vi "CR-SaveImageCCD3暂存.vi"(6 "类型":string(combo)="Front conveyor", 8 "error in (no error)":errorcluster, 9 "Image in":T1(plugin-control), 10 "布尔":bool=TRUE, 11 "基路径":path) -> (0 "error out":errorcluster)   [LabVIEW 2017]
panel:
  out "日期/时间字符串":string
  in  "CCD Name":string(combo)="CCD3"
  out "连接的字符串":string
  # "D:\\Data\\History Image\\20190228\\CCD3\\Image"
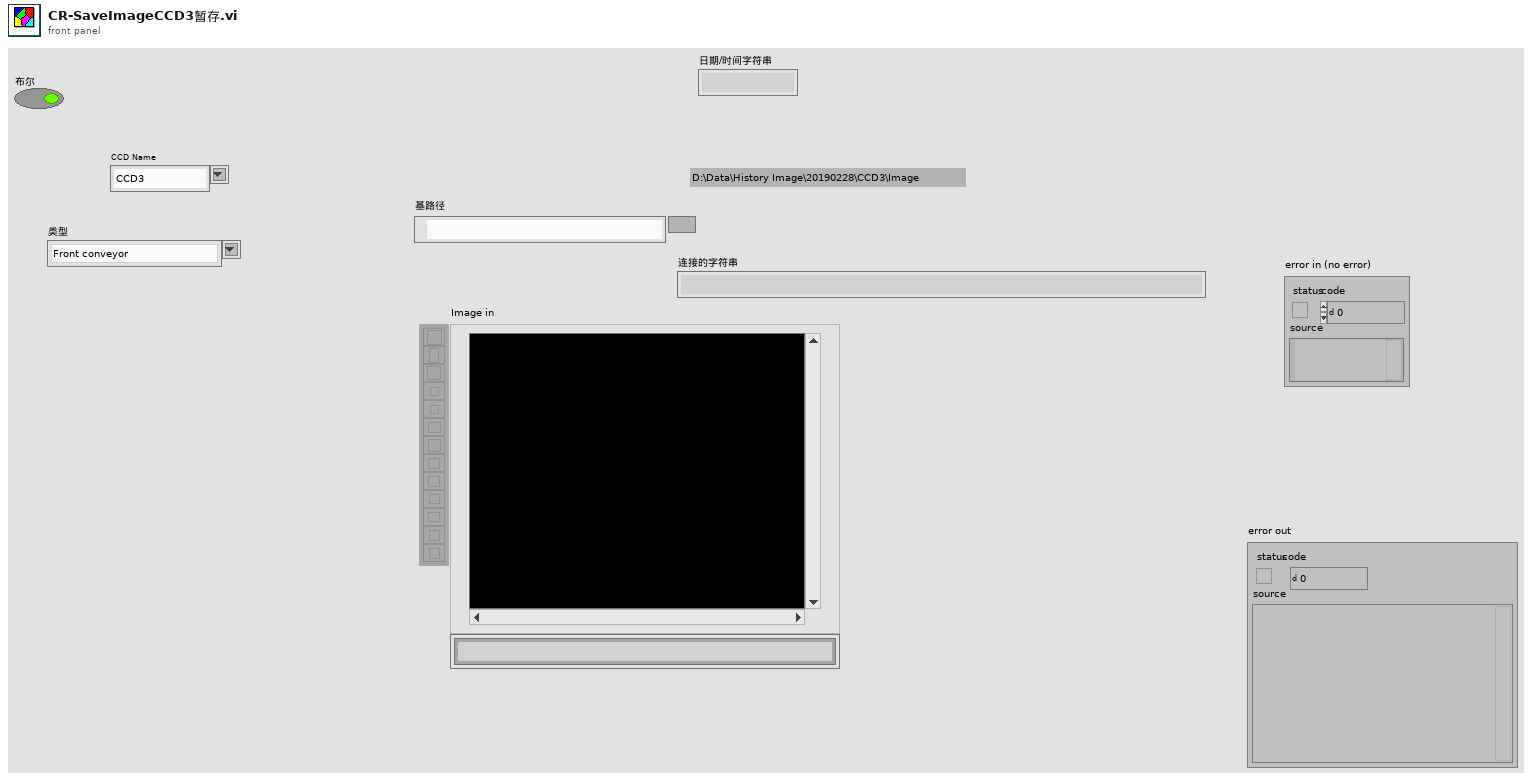
[diagram p1: front panel]
types:
  T1 = typedef "IMAQ Image.ctl" = refnum<image>
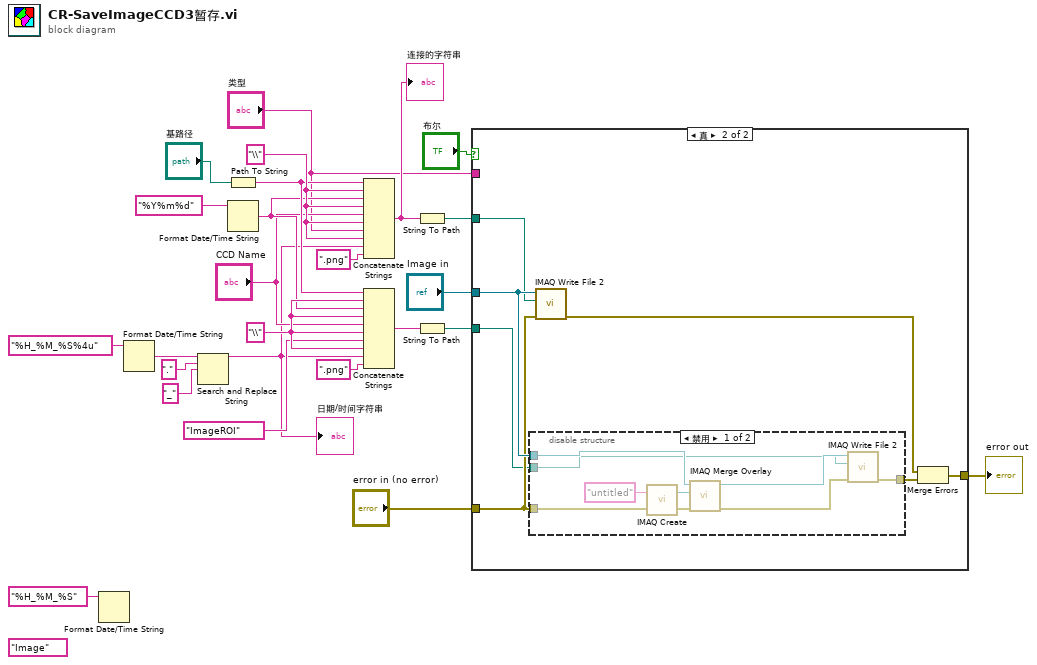
[diagram p0: block diagram]
diagram:
  (unwired) "Image" ("类型")
  w14 = "\\" ("字符串")
  w17 = "\\" ("字符串")
  n1 = Format Date/Time String(time format string (%c)="%H_%M_%S" ("时间格式字符串(%c)")) -> ()  [unwired: 2 in, 1 out]
  n2 = Format Date/Time String(time format string (%c)="%H_%M_%S%4u" ("时间格式字符串(%c)")) -> (date/time string=w4:string)  [unwired: 2 in]
  n3 = Search and Replace String(input string=w4, search string="." ("搜索字符串"), replace string="_" ("替换字符串(\"\")")) -> (result string=w1:string)  [unwired: 5 in, 3 out]
  "日期/时间字符串" <- w1
  n4 = Path To String(path="基路径") -> (string=w12:string)
  n5 = Format Date/Time String(time format string (%c)="%Y%m%d" ("时间格式字符串(%c)")) -> (date/time string=w11:string)  [unwired: 2 in]
  n6 = Concatenate Strings(w12, w17, w11, w17, "CCD Name", w17, "类型", w17, w1, ".png" ("字符串")) -> (w23:string)
  "连接的字符串" <- w23
  n7 = Concatenate Strings(w12, w14, w11, w14, "CCD Name", w14, "ImageROI" ("类型"), w14, w1, ".png" ("字符串")) -> (w8:string)
  n8 = String To Path(string=w23) -> (path=w19:path)
  n9 = String To Path(string=w8) -> (path=w7:path)
  n10 = case shown="真" "布尔" {
    tunnel: "Image in" -> [_ w33]
    tunnel: "error in (no error)" -> [w26 w32]
    tunnel: w19 -> [_ w27]
    tunnel: [w26 w29] -> w16
    tunnel: "类型" -> [_ _]
    tunnel: w7 -> [_ w28]
    frame False {
    }
    frame True {
      n11 = disable-structure shown="禁用" {
        disable-tunnel: w33 -> [w42 _]
        disable-tunnel: w32 -> [w41 _]
        disable-tunnel: [w35 _] -> w31
        disable-tunnel: w28 -> [w34 _]
        frame Disabled {
          n12 = call "IMAQ Create"("Image Name"="untitled", "error in (no error)"=w41) -> ("New Image"=w37:T1, "error out"=w36:errorcluster)  [unwired: 3 in]
          n13 = call "IMAQ Merge Overlay"("error in (no error)"=w36, "Image Dst"=w37, "Image Src"=w42) -> ("error out"=w39:errorcluster, "Image Dst Out"=w40:T1)  [unwired: 7 in]
          n14 = call-poly "IMAQ Write File 2"("error in (no error)"=w39, "File Path"=w34, "Image"=w40) -> ("error out"=w35:errorcluster)  [unwired: 7 in, 1 out]
        }
        frame Enabled {
        }
      }
      n15 = call-poly "IMAQ Write File 2"("error in (no error)"=w32, "File Path"=w27, "Image"=w33) -> ("error out"=w30:errorcluster)  [unwired: 7 in, 1 out]
      n16 = Merge Errors(w30, w31) -> (w29:errorcluster)
    }
  }
  "error out" <- w16
